vi "Add ECU Event Measurement RTM.vi"(8 "error in (no error)":errorcluster, 11 "Node Ptr":u64 format="%.0x") -> (0 "error out":errorcluster)   [LabVIEW 2011, in "Engine Sim System Explorer.lvlib"]
uses:
  Engine Sim System Explorer.lvlib
  <vilib>/NI Veristand/Custom Device API/Custom Device Channel.ctl
  <vilib>/NI Veristand/Custom Device API/Custom Device Channel Type.ctl
  Shared/Engine Simulation Global.vi
  <vilib>/NI Veristand/Custom Device API/Get Item Property (Variant).vi
  Engine Simulation Shared.lvlib
  <vilib>/NI Veristand/Custom Device Tools/Custom Device Utility Library/Custom Device Utility Library.lvlib
  <vilib>/NI Veristand/Custom Device API/Custom Device API.lvlib
panel:
  in  "Tag":string
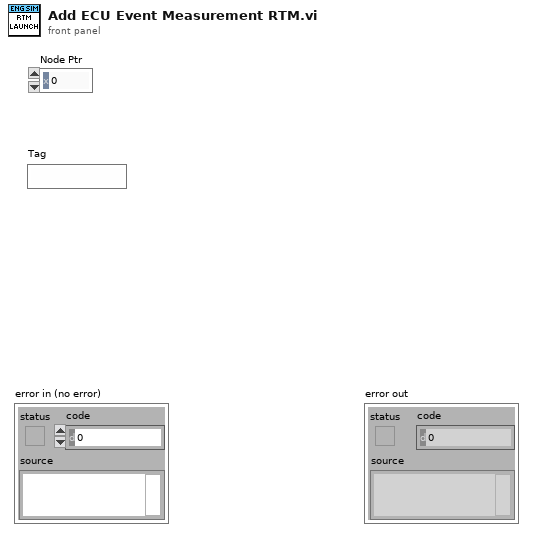
[diagram p1: front panel]
types:
  T1 = typedef "Custom Device API.lvlib/Custom Device Channel.ctl" = cluster{"Type":T2, "Units":string, "Default Value":dbl, "Faultable":bool, "Scalable":bool}
  T2 = typedef "Custom Device API.lvlib/Custom Device Channel Type.ctl" = enum16{"Input", "Output"}
  T3 = cluster{"Time Duration":bool, "Start Angle":bool, "End Angle":bool, "Angle Duration":bool}
  T4 = typedef "Custom Device API.lvlib/Custom Device Item Info.ctl" = cluster{"Name":string, "Is Channel":bool, "GUID":string}
  T5 = typedef "Custom Device API.lvlib/Custom Device Item Ref.ctl" = u64
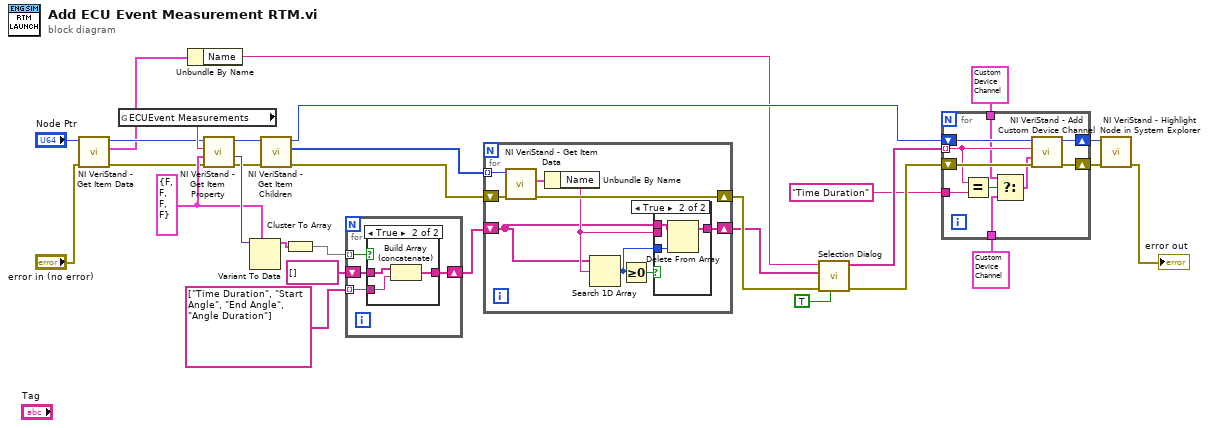
[diagram p0: block diagram]
diagram:
  w25 = T3 {"Time Duration"=FALSE, "Start Angle"=FALSE, "End Angle"=FALSE, "Angle Duration"=FALSE}
  n1 = call <vilib>:"NI VeriStand - Get Item Data.vi"("error in (no error)"="error in (no error)", "Item Ref in"="Node Ptr") -> ("error out"=w10:errorcluster, "Item Info"=w7:T4, "Item Ref out"=w8:T5)  [unwired: 6 in, 1 out]
  n2 = global read "Engine Simulation Global.vi" "ECUEvent Measurements"() -> (w27:string)
  n3 = Unbundle By Name(w7) -> ("Name"=w6:string)
  n4 = call-poly <vilib>:"NI VeriStand - Get Item Property.vi"("error in (no error)"=w10, "Default Value"=w25, "Property Name"=w27, "Item Ref in"=w8) -> ("error out"=w19:errorcluster, "Value"=w26:variant, "Item Ref out"=w18:T5)  [unwired: 4 in, 1 out]
  n5 = Variant To Data(type=w25, Variant=w26) -> (data=w24:T3)  [unwired: 1 in, 1 out]
  n6 = call <vilib>:"NI VeriStand - Get Item Children.vi"("error in (no error)"=w19, "Item Ref in"=w18) -> ("error out"=w4:errorcluster, "Child Refs"=w5:T5[], "Item Ref out"=w15:T5)  [unwired: 6 in, 1 out]
  n7 = Cluster To Array(cluster=w24) -> (array=w23:bool[])
  n8 = for {
    tunnel: w23 -> [w34] mode=indexing
    tunnel: string[] ["Time Duration", "Start Angle", "End Angle", "Angle Duration"] -> [w33] mode=indexing
    shift-right: [w32] -> w1
    shift-left: string[] [] -> [w31]
    n9 = case shown="True" w34 {
      tunnel: w33 -> [_ w38]
      tunnel: [w35 w37] -> w32
      tunnel: w31 -> [w35 w36]
      frame False {
      }
      frame True {
        n10 = Build Array (concatenate)(w36, w38) -> (w37:string[])
      }
    }
  }
  n11 = for {
    tunnel: w5 -> [w47] mode=indexing
    shift-right: [w45] -> w3
    shift-left: w4 -> [w44]
    shift-right: [w42] -> w2
    shift-left: w1 -> [w40]
    n12 = call <vilib>:"NI VeriStand - Get Item Data.vi"("error in (no error)"=w44, "Item Ref in"=w47) -> ("error out"=w45:errorcluster, "Item Info"=w46:T4)  [unwired: 6 in, 2 out]
    n13 = Unbundle By Name(w46) -> ("Name"=w41:string)
    n14 = Search 1D Array(1D array=w40, element=w41) -> (index of element=w39:i32)  [unwired: 1 in]
    n15 = Greater Or Equal To 0?(x=w39) -> (x >= 0?=w43:bool)
    n16 = case shown="True" w43 {
      tunnel: [w48 w50] -> w42
      tunnel: w41 -> [_ _]
      tunnel: w40 -> [w48 w51]
      tunnel: w39 -> [_ w49]
      frame False {
      }
      frame True {
        n17 = Delete From Array(array=w51, index=w49) -> (array with subset deleted=w50:string[])  [unwired: 1 in, 1 out]
      }
    }
  }
  n18 = call "Selection Dialog.vi"("Multi-Selection?"=TRUE, "error in (no error)"=w3, "Tree Items"=w2, "Root Tag"=w6) -> ("error out"=w16:errorcluster, "Selected Names"=w14:string[])  [unwired: 5 in, 1 out]
  n19 = for {
    shift-right: [w60] -> w29
    shift-left: w16 -> [w59]
    shift-right: [w61] -> w30
    shift-left: w15 -> [w58]
    tunnel: w14 -> [w57] mode=indexing
    tunnel: T1 {"Type"=enum."Output", "Units"="Degrees", "Default Value"=0.0, "Faultable"=FALSE, "Scalable"=FALSE} ("Channel") -> [w54]
    tunnel: "Time Duration" ("y") -> [w56]
    tunnel: T1 {"Type"=enum."Output", "Units"="microsecond", "Default Value"=0.0, "Faultable"=FALSE, "Scalable"=FALSE} ("Channel") -> [w53]
    n20 = Equal?(x=w57, y=w56) -> (x = y?=w55:bool)
    n21 = Select(t=w53, s=w55, f=w54) -> (s? t:f=w52:T1)
    n22 = call <vilib>:"NI VeriStand - Add Custom Device Channel.vi"("error in (no error)"=w59, "Channel"=w52, "Channel Name"=w57, "Parent Ref in"=w58) -> ("error out"=w60:errorcluster, "Parent Ref out"=w61:T5)  [unwired: 4 in, 2 out]
  }
  n23 = call <vilib>:"NI VeriStand - Highlight Node in System Explorer.vi"("error in (no error)"=w29, "Item Ref in"=w30) -> ("error out"=→"error out":errorcluster)  [unwired: 8 in, 1 out]
